vi "CTAH Controller.vi"   [LabVIEW 2017]
uses:
  <vilib>/addons/control/pid/pid.llb/PID (DBL).vi
  <vilib>/addons/control/pid/pid.llb/PID Output Rate Limiter (DBL).vi
  <vilib>/addons/control/pid/NI_PID_pid.lvlib
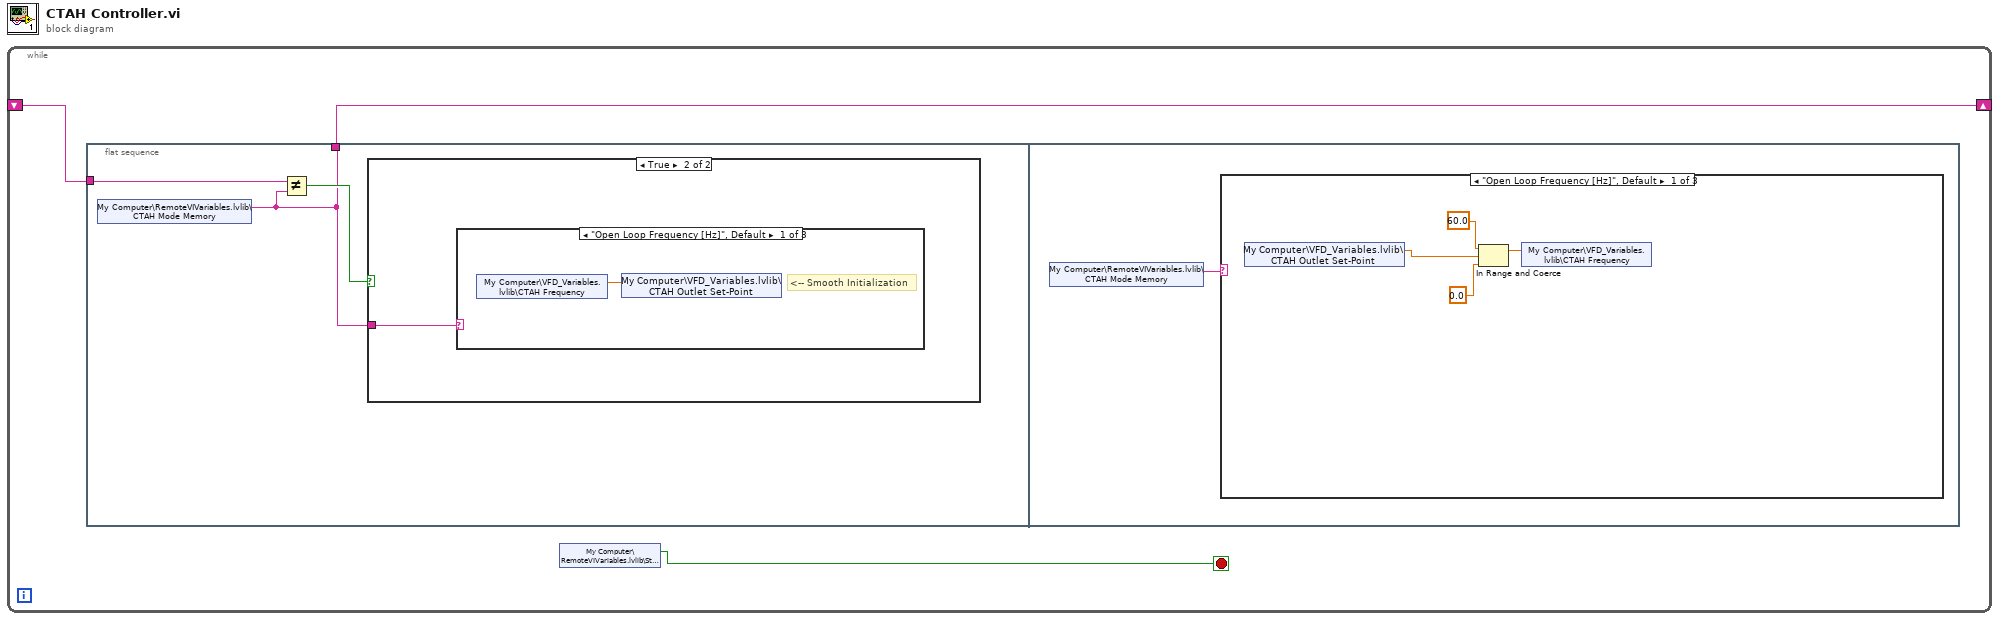
[diagram p0: block diagram]
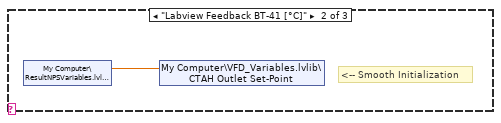
[diagram p3: hidden frame]
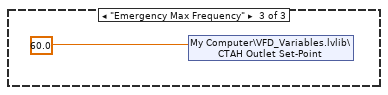
[diagram p4: hidden frame]
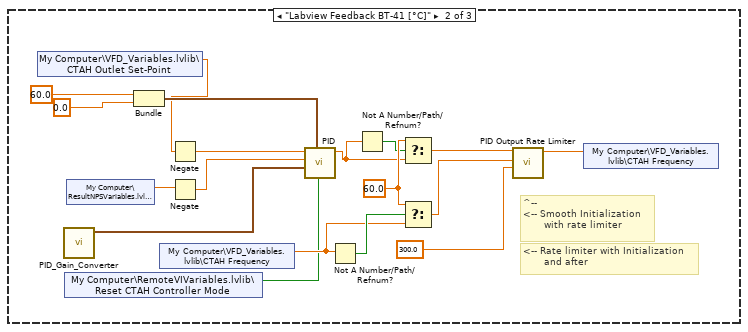
[diagram p5: hidden frame]
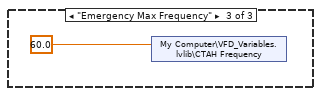
[diagram p6: hidden frame]
diagram:
  n1 = while {
    shift-right: [w1] -> _
    shift-left: _ -> [w2]
    stop <- w3 stop-if-true
    n2 = flat-sequence {
      tunnel: w2 -> [w6]
      tunnel: [w4] -> w1
      frame #0 {
        n3 = shared-variable "My Computer\\RemoteVIVariables.lvlib\\CTAH Mode Memory"() -> (w4:string)  [unwired: 1 in, 1 out]
        n4 = Not Equal?(x=w6, y=w4) -> (x != y?=w5:bool)
        n5 = case shown="True" w5 {
          tunnel: w4 -> [_ w7]
          frame False {
          }
          frame True {
            n6 = case shown="\"Open Loop Frequency [Hz]\", Default" w7 {
              frame "Open Loop Frequency [Hz]", Default {
                # "<-- Smooth Initialization"
                n7 = shared-variable "My Computer\\VFD_Variables.lvlib\\CTAH Frequency"() -> (w8:sgl)  [unwired: 1 in, 1 out]
                n8 = shared-variable "My Computer\\VFD_Variables.lvlib\\CTAH Outlet Set-Point"(w8) -> ()  [unwired: 1 in, 1 out]
              }
              frame "Labview Feedback BT-41 [°C]" {
                # "<-- Smooth Initialization"
                n9 = shared-variable "My Computer\\ResultNPSVariables.lvlib\\BT-41_R"() -> (w9:sgl)  [unwired: 1 in, 1 out]
                n10 = shared-variable "My Computer\\VFD_Variables.lvlib\\CTAH Outlet Set-Point"(w9) -> ()  [unwired: 1 in, 1 out]
              }
              frame "Emergency Max Frequency" {
                n11 = shared-variable "My Computer\\VFD_Variables.lvlib\\CTAH Outlet Set-Point"(60.0) -> ()  [unwired: 1 in, 1 out]
              }
            }
          }
        }
      }
      frame #1 {
        n12 = shared-variable "My Computer\\RemoteVIVariables.lvlib\\CTAH Mode Memory"() -> (w11:string)  [unwired: 1 in, 1 out]
        n13 = case shown="\"Open Loop Frequency [Hz]\", Default" w11 {
          frame "Open Loop Frequency [Hz]", Default {
            n14 = shared-variable "My Computer\\VFD_Variables.lvlib\\CTAH Outlet Set-Point"() -> (w15:dbl)  [unwired: 1 in, 1 out]
            n15 = In Range and Coerce(upper limit=sgl 60.0, x=w15, lower limit=sgl 0.0) -> (coerced(x)=w14:dbl)  [unwired: 1 out]
            n16 = shared-variable "My Computer\\VFD_Variables.lvlib\\CTAH Frequency"(w14) -> ()  [unwired: 1 in, 1 out]
          }
          frame "Labview Feedback BT-41 [°C]" {
            w23 = 60.0
            # "<-- Rate limiter with Initialization\n       and after"
            # "^--\n<-- Smooth Initialization\n       with rate limiter"
            n17 = shared-variable "My Computer\\VFD_Variables.lvlib\\CTAH Outlet Set-Point"() -> (w17:dbl)  [unwired: 1 in, 1 out]
            n18 = call "PID_Gain_Converter.vi"() -> ("Cluster"=w30:cluster{dbl, dbl, dbl})  [unwired: 11 in]
            n19 = shared-variable "My Computer\\RemoteVIVariables.lvlib\\Reset CTAH Controller Mode"() -> (w16:bool)  [unwired: 1 in, 1 out]
            n20 = shared-variable "My Computer\\ResultNPSVariables.lvlib\\BT-41_R"() -> (w18:sgl)  [unwired: 1 in, 1 out]
            n21 = Bundle(60.0, 0.0) -> (w33:cluster{dbl, dbl})  [unwired: 1 in]
            n22 = shared-variable "My Computer\\VFD_Variables.lvlib\\CTAH Frequency"() -> (w26:sgl)  [unwired: 1 in, 1 out]
            n23 = Negate(x=w17) -> (-x=w20:dbl)
            n24 = Negate(x=w18) -> (-x=w19:sgl)
            n25 = call-poly <vilib>:"PID.vi"("reinitialize? (F)"=w16, "output range"=w33, "PID gains"=w30, "process variable"=w19, "setpoint"=w20) -> ("output"=w21:dbl)  [unwired: 5 in, 1 out]
            n26 = Not A Number/Path/Refnum?(number/path/refnum=w26) -> (NaN/Path/Refnum?=w27:bool)
            n27 = Not A Number/Path/Refnum?(number/path/refnum=w21) -> (NaN/Path/Refnum?=w22:bool)
            n28 = Select(t=w23, s=w22, f=w21) -> (s? t:f=w24:dbl)
            n29 = Select(t=w23, s=w27, f=w26) -> (s? t:f=w25:dbl)
            n30 = call-poly <vilib>:"PID Output Rate Limiter.vi"("output rate (EGU/min)"=300.0, "initial output"=w25, "input (controller output)"=w24) -> ("output"=w29:dbl)  [unwired: 5 in, 1 out]
            n31 = shared-variable "My Computer\\VFD_Variables.lvlib\\CTAH Frequency"(w29) -> ()  [unwired: 1 in, 1 out]
          }
          frame "Emergency Max Frequency" {
            n32 = shared-variable "My Computer\\VFD_Variables.lvlib\\CTAH Frequency"(60.0) -> ()  [unwired: 1 in, 1 out]
          }
        }
      }
    }
    n33 = shared-variable "My Computer\\RemoteVIVariables.lvlib\\Stop CTAH"() -> (w3:bool)  [unwired: 1 in, 1 out]
  }
